vi "cubo.vi"() -> ()   [LabVIEW 2016]
panel:
  out "new picture 6":picture
  in  "3 1":dbl(slide) scale=0.0..255.0
  out "new picture 5":picture
  in  "2 1":dbl(slide) scale=0.0..255.0
  out "new picture 4":picture
  in  "12":dbl(slide) scale=0.0..255.0
  out "new picture 3":picture
  in  "3":dbl(slide) scale=0.0..255.0
  in  "2":dbl(slide) scale=0.0..255.0
  out "new picture 2":picture
  in  "1":dbl(slide) scale=0.0..255.0
  out "new picture":picture
  # "(255)"
  # "(0)"
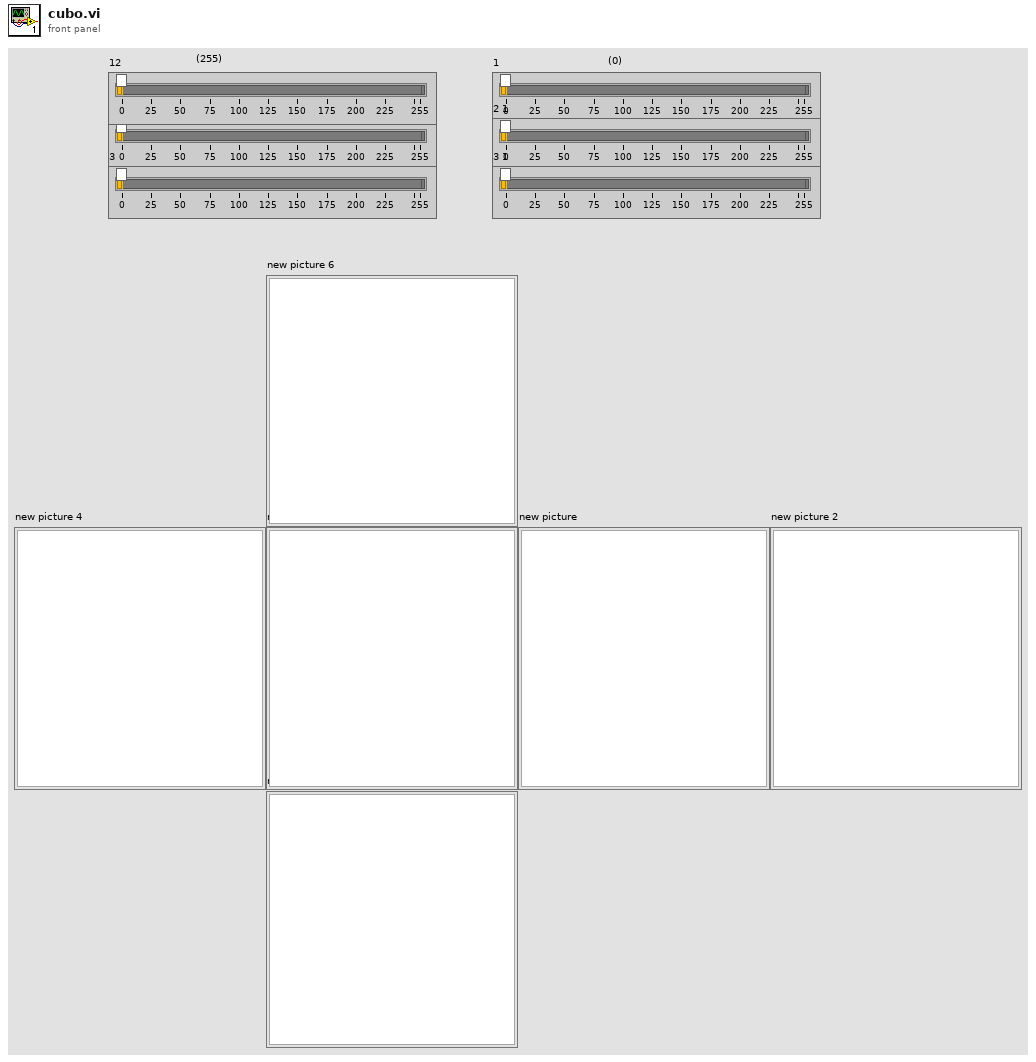
[diagram p1: front panel]
types:
  T1 = typedef "imagedata.ctl" = cluster{"image type":i32, "image depth":i32, "image":u8[], "mask":u8[], "colors":u32[], "Rectangle":cluster{"left":i16, "top":i16, "right":i16, "bottom":i16}}
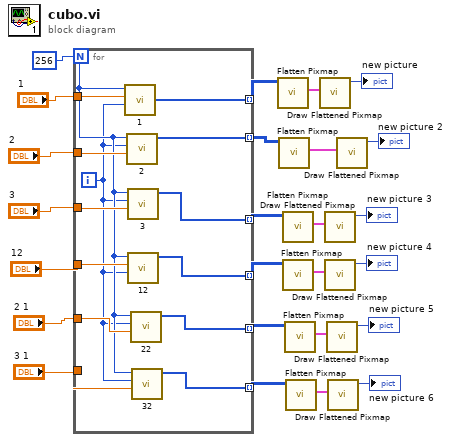
[diagram p0: block diagram]
diagram:
  n1 = for {
    N: 256 -> [w27]
    tunnel: [w39] -> w24 mode=indexing
    tunnel: "1" -> [w38]
    tunnel: [w37] -> w18 mode=indexing
    tunnel: "2" -> [w36]
    tunnel: "3" -> [w35]
    tunnel: [w34] -> w13 mode=indexing
    tunnel: "12" -> [w33]
    tunnel: [w32] -> w9 mode=indexing
    tunnel: "2 1" -> [w31]
    tunnel: [w30] -> w5 mode=indexing
    tunnel: "3 1" -> [w29]
    tunnel: [w28] -> w1 mode=indexing
    i -> [w26]
    n2 = call "1.vi"("Numeric"=w26, "1"=w38, "Numeric 2"=w27) -> ("Array"=w39:u32[])  [unwired: 8 in]
    n3 = call "2.vi"("2"=w36, "Numeric"=w26, "Numeric 2"=w27) -> ("Array"=w37:u32[])  [unwired: 8 in]
    n4 = call "3.vi"("3"=w35, "Numeric"=w26, "Numeric 2"=w27) -> ("Array"=w34:u32[])  [unwired: 8 in]
    n5 = call "12.vi"("Numeric"=w26, "1"=w33, "Numeric 2"=w27) -> ("Array"=w32:u32[])  [unwired: 8 in]
    n6 = call "22.vi"("2"=w31, "Numeric"=w26, "Numeric 2"=w27) -> ("Array"=w30:u32[])  [unwired: 8 in]
    n7 = call "32.vi"("3"=w29, "Numeric"=w26, "Numeric 2"=w27) -> ("Array"=w28:u32[])  [unwired: 8 in]
  }
  n8 = call <vilib>:"Flatten Pixmap.vi"("24-bit pixmap"=w24) -> ("image data"=w23:T1)  [unwired: 10 in]
  n9 = call <vilib>:"Flatten Pixmap.vi"("24-bit pixmap"=w18) -> ("image data"=w20:T1)  [unwired: 10 in]
  n10 = call <vilib>:"Flatten Pixmap.vi"("24-bit pixmap"=w13) -> ("image data"=w14:T1)  [unwired: 10 in]
  n11 = call <vilib>:"Flatten Pixmap.vi"("24-bit pixmap"=w9) -> ("image data"=w11:T1)  [unwired: 10 in]
  n12 = call <vilib>:"Flatten Pixmap.vi"("24-bit pixmap"=w5) -> ("image data"=w6:T1)  [unwired: 10 in]
  n13 = call <vilib>:"Flatten Pixmap.vi"("24-bit pixmap"=w1) -> ("image data"=w3:T1)  [unwired: 10 in]
  n14 = call <vilib>:"Draw Flattened Pixmap.vi"("image data"=w23) -> ("new picture"=→"new picture":picture)  [unwired: 8 in]
  n15 = call <vilib>:"Draw Flattened Pixmap.vi"("image data"=w14) -> ("new picture"=→"new picture 3":picture)  [unwired: 8 in]
  n16 = call <vilib>:"Draw Flattened Pixmap.vi"("image data"=w11) -> ("new picture"=→"new picture 4":picture)  [unwired: 8 in]
  n17 = call <vilib>:"Draw Flattened Pixmap.vi"("image data"=w6) -> ("new picture"=→"new picture 5":picture)  [unwired: 8 in]
  n18 = call <vilib>:"Draw Flattened Pixmap.vi"("image data"=w3) -> ("new picture"=→"new picture 6":picture)  [unwired: 8 in]
  n19 = call <vilib>:"Draw Flattened Pixmap.vi"("image data"=w20) -> ("new picture"=→"new picture 2":picture)  [unwired: 8 in]
